vi "Read Analog Input.vi"(8 "error in (no error)":errorcluster, 10 "Channel":i32, 11 "VISA resource name in":refnum<visa-resource-name>) -> (0 "error out":errorcluster, 1 "Value":u16, 3 "VISA resource name":refnum<visa-resource-name>)   [LabVIEW 2020, in "CTI-Visa.lvlib"]
uses:
  CTI-Visa.lvlib
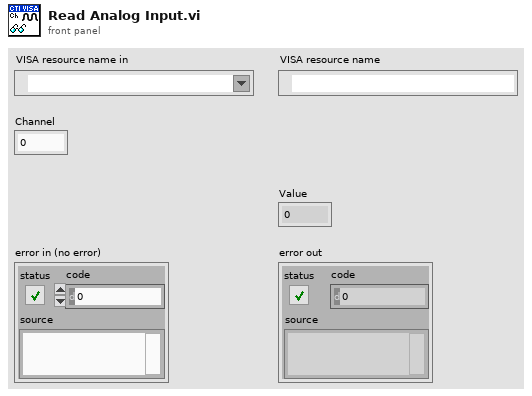
[diagram p1: front panel]
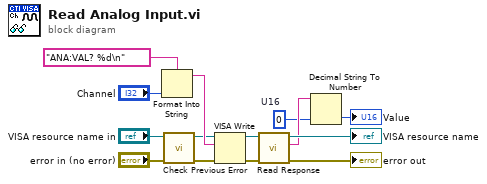
[diagram p0: block diagram]
diagram:
  w8 = u16 0  # U16
  n1 = Format Into String(format string="ANA:VAL? %d\n", "Channel") -> (resulting string=w13:string)  [unwired: 2 in, 1 out]
  n2 = call "Check Previous Error.vi"("error in (no error)"="error in (no error)", "VISA resource name in"="VISA resource name in") -> ("error out"=w1:errorcluster, "VISA resource name"=w3:refnum<visa-resource-name>)  [unwired: 8 in]
  n3 = VISA Write(VISA resource name=w3, write buffer=w13, error in (no error)=w1) -> (VISA resource name out=w4:refnum<visa-resource-name>, error out=w12:errorcluster)  [unwired: 1 out]
  n4 = call "Read Response.vi"("error in (no error)"=w12, "VISA resource name in"=w4) -> ("error out"=→"error out":errorcluster, "Response"=w9:string, "VISA resource name"=→"VISA resource name":refnum<visa-resource-name>)  [unwired: 7 in]
  n5 = Decimal String To Number(string=w9, default (0L)=w8) -> (number=→"Value":u16)  [unwired: 1 in, 1 out]
